vi "CSM Example - Caller is a CSM.vi"() -> ()   [LabVIEW 2017]
doc: "### CSM Example - Caller is a CSM.vi\n\n#### Overview\n\nDemonstrates how to invoke CSM module within the CSM framework. In this example, inter-module communication is performed through message string queue operations. You can generate a message string using the Build Message with Arguments++ VI or directly use message description strings if you are familiar with the format.\n\nThis example synchronously calls two instances of CSM Reuse Module.vi, enabling dynamic status subscription and module control through the API.\n\n#### Introduction\n\nDemonstrates how to invoke CSM module within the CSM framework. In this example, inter-module communication is performed through message string queue operations. You can generate a message string using the Build Message with Arguments++ VI or directly use message description strings if you are familiar with the format.\n\nThis example synchronously calls two instances of CSM Reuse Module.vi, enabling dynamic status subscription and module control through the API.\n\n#### Steps\n\nStep 1: Drop a VI CSM UI Module Template from LabVIEW palette, change the CSM name to \"CSMScenarioExample\".\n\nStep 2: Synchronously call the CSM Reuse Module.vi twice and name them SubModule0 and SubModule1 respectively. For more details of how to create such a reuse CSM module, please refer to another CSM-example named 1. Create a reuse Module.\n\nStep 3: Add one new line of customized message string, namely \"Macro: Switch Active Module\" as the last line into the existing standard string queues under \"Macro:Initialize\" case, so that we can switch between different SubModules.\n\nStep 4: Add one string constant SubModule0 for internal data initialization. For more customized internal data initialization, we can add more code here. \n\nStep 5: Add one string control in the UI to switch and display active/target module (Combox box).\n Step 5.1: Under \" 'Target Module': Value Change\" UI event, set the string control to the active module internal data and also send one intra-module message Macro: Switch Active. Module. \n Step 5.2: Under \"UI: Initialize\" case, update the active/Target Module.\n\nStep 6: Under \"Macro: Switch Active Module\" case, use the high level VI to send an inter-module sync. message \"API: Get Level -@ modulename\" to the active SubModule.\nOr you can also just type the string constant manually if you're familiar with the CSM string syntax rules. \n\nStep 7: Now the status queue is empty and the CSM state machine is now waiting in the timeout UI-event under ' \"\", \"Event Structure\", \"Idle\" '. The next step depends on the UI interaction provided by the User. \n\nStep 8: Create local test buttons/controls in the UI as follows:\n Step 8.1: Create API:Start button, when user clicks this button, a async-No reply message, \"API: Start -> modulename\" will be send to start the active subModule. \n Step 8.2: Create Register All Status Change button, when user clicks this button, this CSM module registers following broadcast/interrupt message from the active SubModule \n\"Status Changed@* >> Action: Status Change Handler -><register>\".\n Step 8.3: Create Unregister All Status Change button, when user clicks this button, this CSM module unregisters following broadcast/interrupt message from the active SubModule \n\"Status Changed@* >> Action: Status Change Handler -><unregister>\".\n Step 8.4: No code here, but you can see the log when it's called because of the registered status change. Any further customized code can be added here right after receiving this broadcast/interrupt message.\n Step 8.5: Create API:Stop button, when user clicks this button, an async-No reply message, \"API: Stop -> modulename\" will be sent to stop the active subModule. \n Step 8.6: Create Level DBL control, when user changes the value, an async message, \"API: Set Level >> 0.3 ->| modulename\" will be sent to the active subModule.\n Step 8.7: Create API: Get Level(Async) button, when user clicks this button, an async message, \"API: Get Level -> modulename\" will be sent to the active SubModule. Handle the case \"Async Message Posted\" and \"Async Response\" accordingly, in this example the Level display will be updated. \n Step 8.8: Create UI: create Front Panel State >> Open button, when user clicks the button, an async message with no reply \"UI: Front Panel State >> Open ->| modulename\" will be sent to the active Submodule.\n Step 8.9: Create UI: create Front Panel State >> Close button, when user clicks the button, an async message with no reply \"UI: Front Panel State >> Close ->| modulename\" will be sent to the active Submodule.\n\nStep 9: Under \"Panel Close?\" UI event, add two more new string messages before \"Macro:Exit\": \"Macro: Exit -@ SubModule0\" and \"Macro: Exit -@ SubModule1\", so that we can safely close all the CSM submodules before we finally close the CSM caller/main module."
uses:
  user.lib/_NEVSTOP/Communicable State Machine(CSM)/_Polymophic/Build Asynchronous Message with Arguments.vi
  user.lib/_NEVSTOP/Communicable State Machine(CSM)/_Polymophic/Build No-Reply Asynchronous Message with Arguments.vi
  user.lib/_NEVSTOP/Communicable State Machine(CSM)/_Polymophic/Build Unregister Status Message.vi
  user.lib/_NEVSTOP/Communicable State Machine(CSM)/_Polymophic/Build Register Status Message.vi
  user.lib/_NEVSTOP/Communicable State Machine(CSM)/_Polymophic/Build Synchronous Message with Arguments.vi
  user.lib/_NEVSTOP/Communicable State Machine(CSM)/Communicable State Machine.lvlib
  1. Create a reuse Module/1. Create a reuse Module.lvlib
panel:
  in  "UI: Front Panel State >> Close":bool
  in  "UI: Front Panel State >> Open":bool
  in  "Level":dbl min=0.0 max=1.0 step=0.1
  in  "Target Module":string(combo)="SubModule0"
  in  "API: Stop":bool
  in  "API: Start":bool
  in  "Unregister All Status Change":bool
  in  "Register All Status Change":bool
  in  "API: Get Level(Async)":bool
  out "State History of Main":string
  # "#CSM-Example Overview\n\nDemonstrates how to invoke CSM module within the CSM framework. In this example, inter-module communication is performed through message string queue operations. You can generate a message string using the Build Message with Arguments++ VI or directly use message description strings if you are familiar with the format.\n\nThis example synchronously calls two instances of CSM Reuse Module.vi, enabling dynamic status subscription and module control through the API."
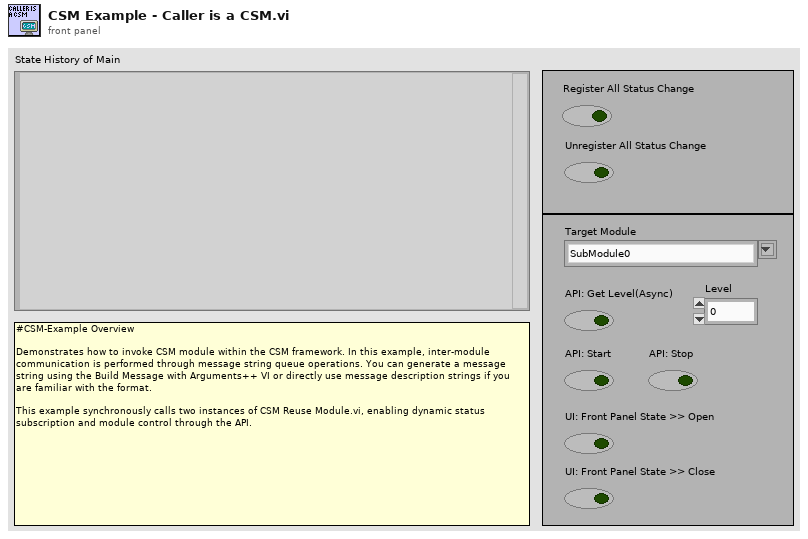
[diagram p1: front panel]
types:
  T1 = enum32{"Invalid", "Standard", "Closed", "Hidden", "Minimized", "Maximized"}
  T2 = enum32{"invalid app kind", "Development System", "Run Time System", "Student Edition", "Embedded LabVIEW", "Evaluation", "Custom"}
  T3 = typedef "Communicable State Machine.lvlib/_CSM_Response Source Message.ctl" = cluster{"‘State":string, "’Arguments":string, "’Error":errorcluster}
  T4 = cluster{"Core":cluster{"Current VI Reference":refnum<vi>, "Close Panel on Exit?":bool}, "Active Module":string}
  T5 = cluster{"Current VI Reference":refnum<vi>, "Close Panel on Exit?":bool}
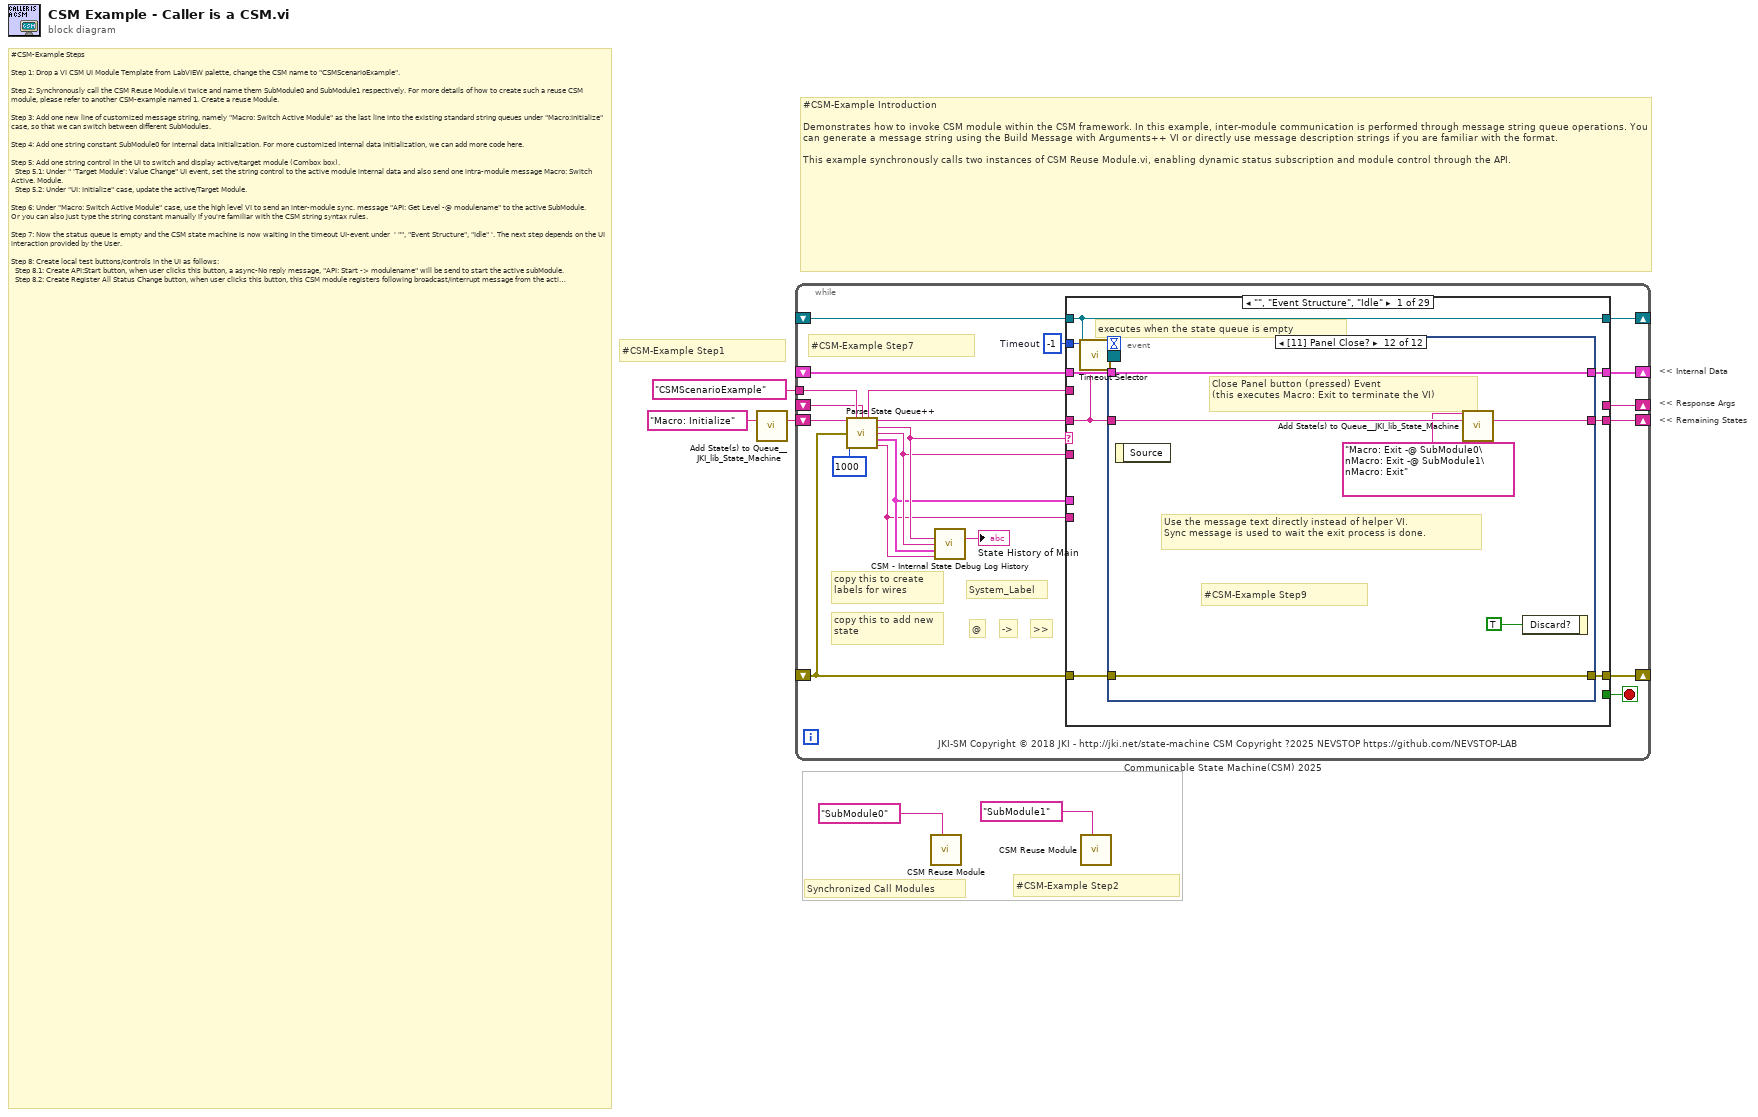
[diagram p0: block diagram]
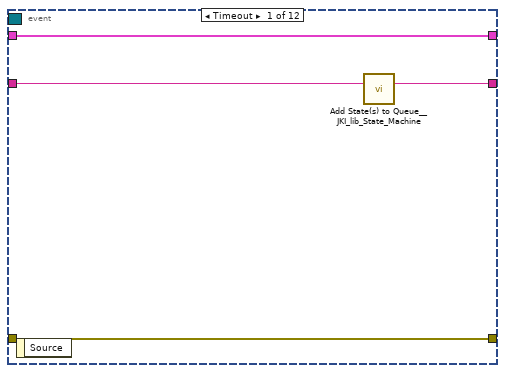
[diagram p2: hidden frame]
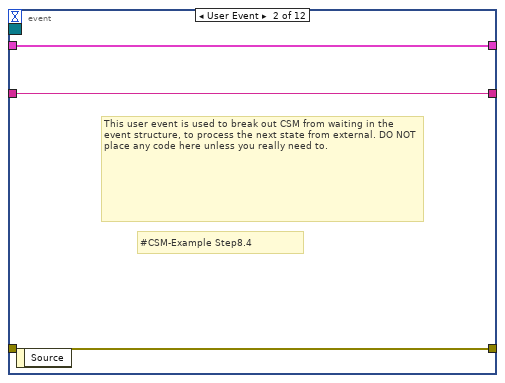
[diagram p3: hidden frame]
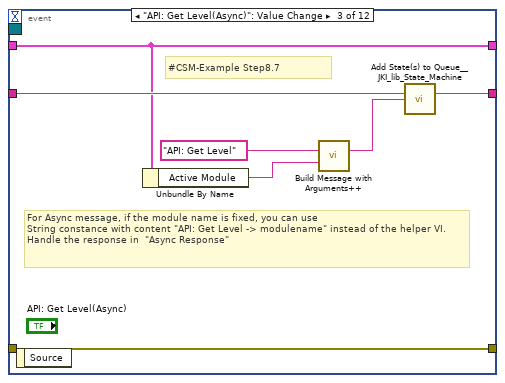
[diagram p4: hidden frame]
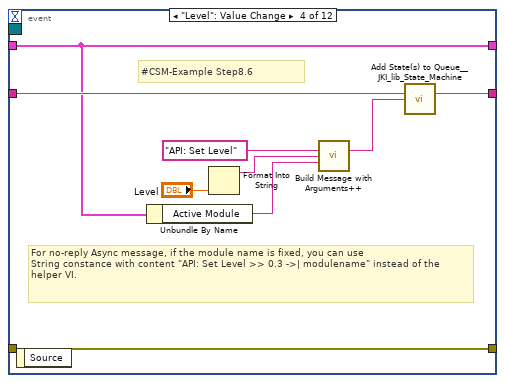
[diagram p5: hidden frame]
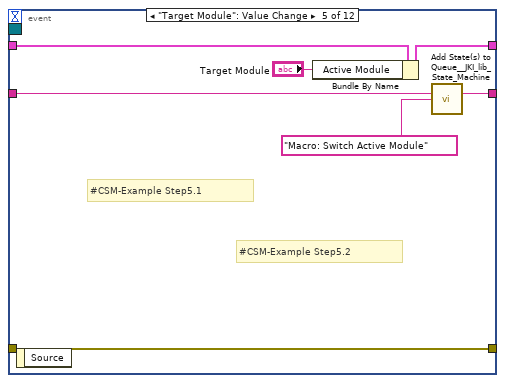
[diagram p6: hidden frame]
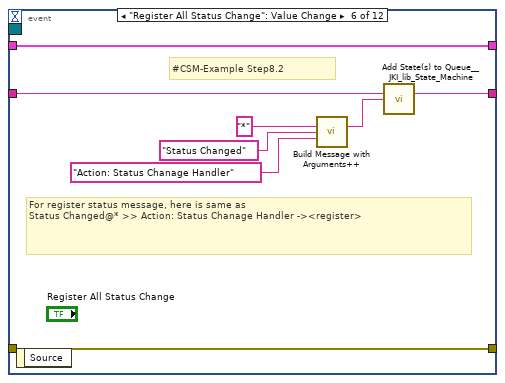
[diagram p7: hidden frame]
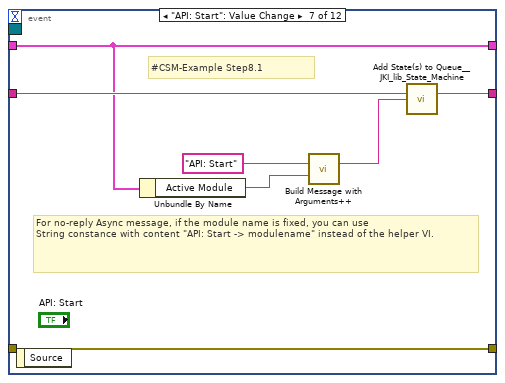
[diagram p8: hidden frame]
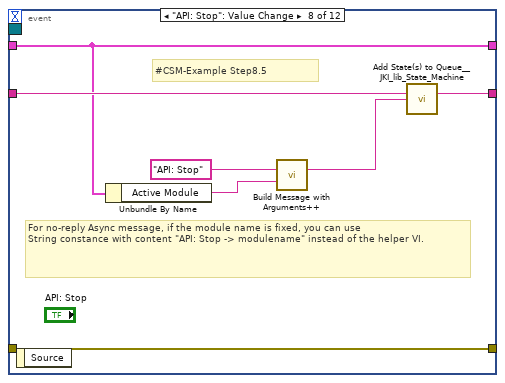
[diagram p9: hidden frame]
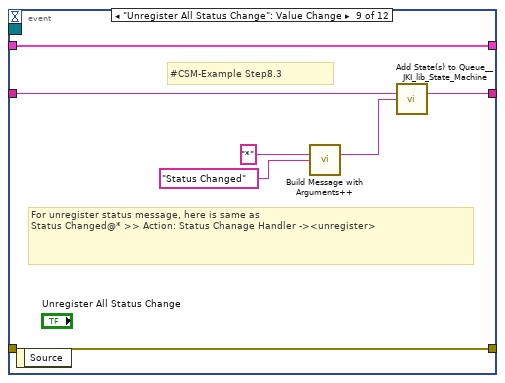
[diagram p10: hidden frame]
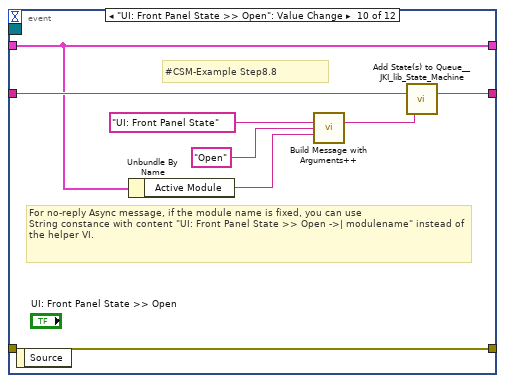
[diagram p11: hidden frame]
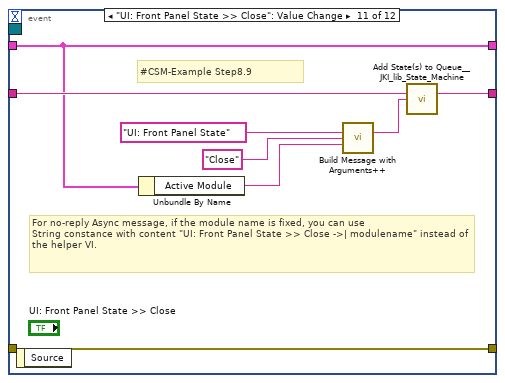
[diagram p12: hidden frame]
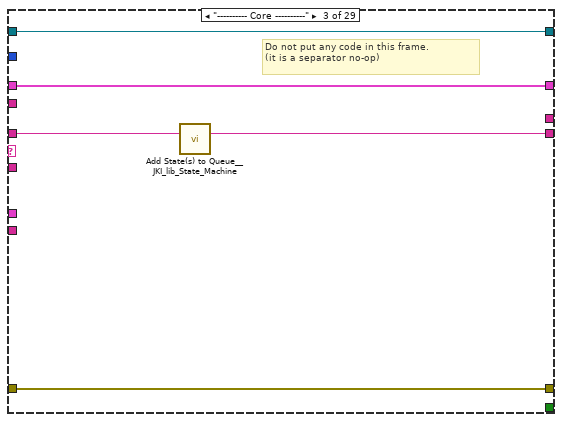
[diagram p14: hidden frame]
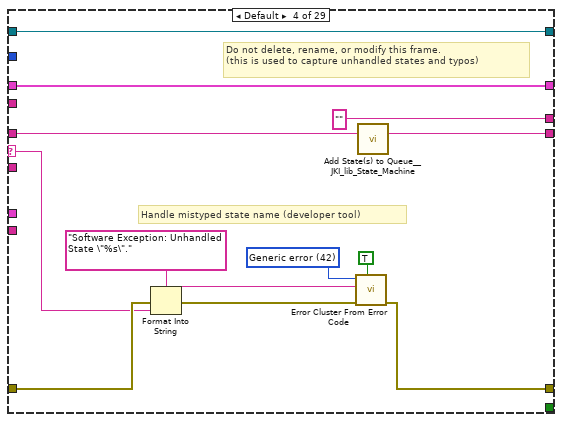
[diagram p15: hidden frame]
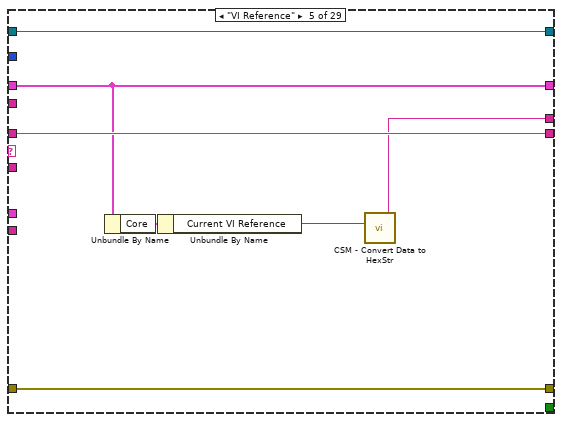
[diagram p16: hidden frame]
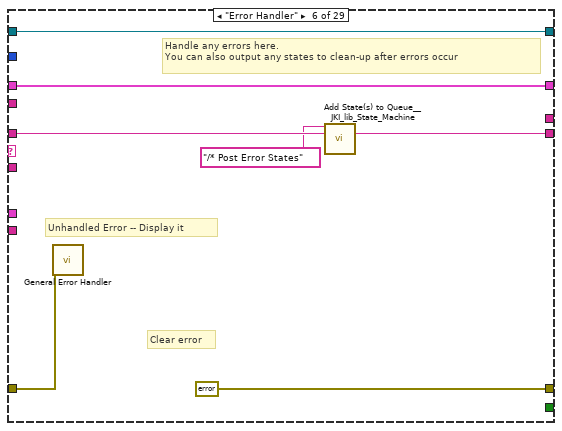
[diagram p17: hidden frame]
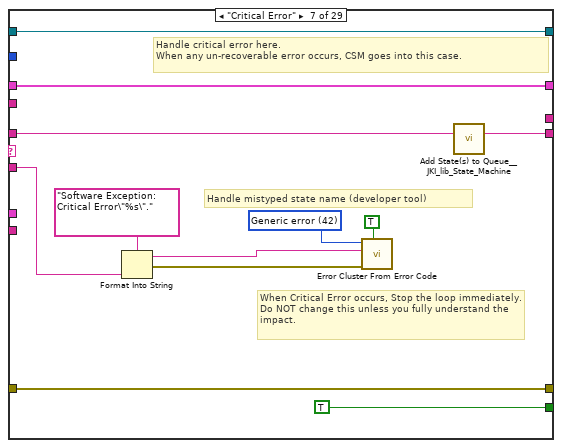
[diagram p18: hidden frame]
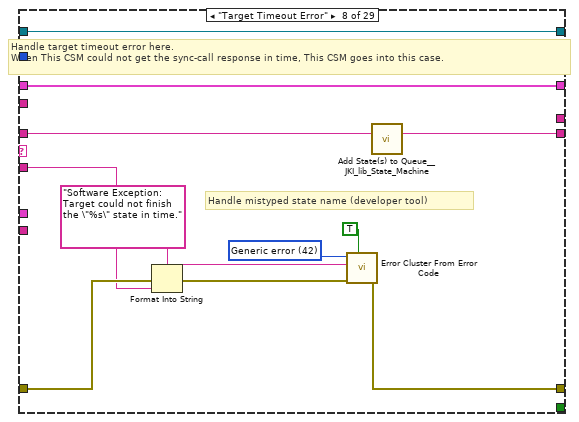
[diagram p19: hidden frame]
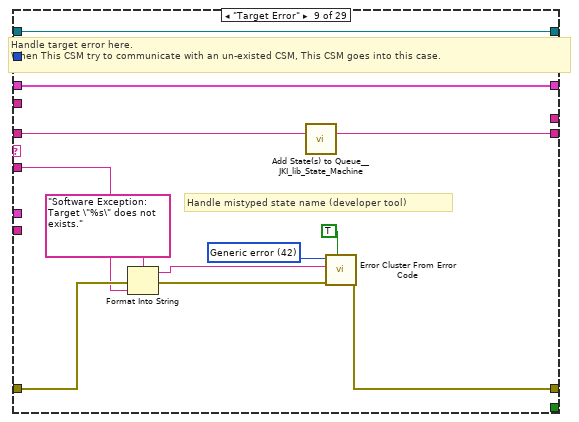
[diagram p20: hidden frame]
diagram:
  # "#CSM-Example Step2"
  # "#CSM-Example Step1"
  # "#CSM-Example Introduction\n\nDemonstrates how to invoke CSM module within the CSM framework. In this example, inter-module communication is performed through message string queue operations. You can generate a message string using the Build Message with Arguments++ VI or directly use message description strings if you are familiar with the format.\n\nThis example synchronously calls two instances of CSM Reuse Module.vi, enabling dynamic status subscription and module control through the API."
  # "#CSM-Example Steps\n\nStep 1: Drop a VI CSM UI Module Template from LabVIEW palette, change the CSM name to \"CSMScenarioExample\".\n\nStep 2: Synchronously call the CSM Reuse Module.vi twice and name them SubModule0 and SubModule1 respectively. For more details of how to create such a reuse CSM module, please refer to another CSM-example named 1. Create a reuse Module.\n\nStep 3: Add one new line of customized message string, namely \"Macro: Switch Active Module\" as the last line into the existing standard string queues under \"Macro:Initialize\" case, so that we can switch between different SubModules.\n\nStep 4: Add one string constant SubModule0 for internal data initialization. For more customized internal data initialization, we can add more code here. \n\nStep 5: Add one string control in the UI to switch and display active/target module (Combox box).\n  Step 5.1: Under \" 'Target Module': Value Change\" UI event, set the string control to the active module internal data and also send one intra-module message Macro: Switch Active. Module. \n  Step 5.2: Under \"UI: Initialize\" case, update the active/Target Module.\n\nStep 6: Under \"Macro: Switch Active Module\" case, use the high level VI to send an inter-module sync. message \"API: Get Level -@ modulename\" to the active SubModule.\nOr you can also just type the string constant manually if you're familiar with the CSM string syntax rules. \n\nStep 7: Now the status queue is empty and the CSM state machine is now waiting in the timeout UI-event under  ' \"\", \"Event Structure\", \"Idle\" '. The next step depends on the UI interaction provided by the User. \n\nStep 8: Create local test buttons/controls in the UI as follows:\n  Step 8.1: Create API:Start button, when user clicks this button, a async-No reply message, \"API: Start -> modulename\" will be send to start the active subModule. \n  Step 8.2: Create Register All Status Change button, when user clicks this button, this CSM module registers following broadcast/interrupt message from the active SubModule \n\"Status Changed@* >> Action: Status Change Handler -><register>\".\n  Step 8.3:  Create Unregister All Status Change button, when user clicks this button, this CSM module unregisters following broadcast/interrupt message from the active SubModule \n\"Status Changed@* >> Action: Status Change Handler -><unregister>\".\n  Step 8.4: No code here, but you can see the log when it's called because of the registered status change. Any further customized code can be added here right after receiving this broadcast/interrupt message.\n  Step 8.5: Create API:Stop button, when user clicks this button, an async-No reply message, \"API: Stop -> modulename\" will be sent to stop the active subModule. \n  Step 8.6: Create Level DBL control, when user changes the value, an async message, \"API: Set Level >> 0.3 ->| modulename\" will be sent to the active subModule.\n  Step 8.7: Create API: Get Level(Async) button, when user clicks this button, an async message, \"API: Get Level -> modulename\" will be sent to the active SubModule. Handle the case \"Async Message Posted\" and \"Async Response\" accordingly, in this example the Level display will be updated.  \n  Step 8.8: Create UI: create Front Panel State >> Open button, when user clicks the button, an async message with no reply \"UI: Front Panel State >> Open ->| modulename\" will be sent to the active Submodule.\n  Step 8.9: Create UI: create Front Panel State >> Close button, when user clicks the button, an async message with no reply \"UI: Front Panel State >> Close ->| modulename\" will be sent to the active Submodule.\n\nStep 9: Under \"Panel Close?\" UI event, add two more new string messages before \"Macro:Exit\": \"Macro: Exit -@ SubModule0\" and \"Macro: Exit -@ SubModule1\", so that we can safely close all the CSM submodules before we finally close the CSM caller/main module."
  # "Synchronized Call Modules"
  # "<< Internal Data"
  # "<< Response Args"
  # "<< Remaining States"
  n1 = call <vilib>:"Add State(s) to Queue__JKI_lib_State_Machine.vi"("State(s) in (\"\")"="Macro: Initialize") -> ("States Out"=w5:string)  [unwired: 14 in]
  n2 = while "Communicable State Machine(CSM) 2025" {
    shift-right: [w21] -> _
    shift-left: _ -> [w20]
    shift-right: [w24] -> _
    shift-left: _ -> [w18]
    shift-right: [w23] -> _
    shift-left: w5 -> [w25]
    tunnel: "CSMScenarioExample" ("Name (\"\" to Use UUID)") -> [w13]
    shift-right: [w16] -> _
    shift-left: _ -> [w7]
    shift-right: [w15] -> _
    shift-left: _ -> [w14]
    stop <- w22 stop-if-true
    w19 = -1  # Timeout
    # "#CSM-Example Step7"
    # "JKI-SM Copyright © 2018 JKI - http://jki.net/state-machine CSM Copyright ?2025 NEVSTOP https://github.com/NEVSTOP-LAB"
    # "copy this to add new state"
    # ">>"
    # "->"
    # "@"
    # "copy this to create labels for wires"
    # "System_Label"
    n3 = call "Parse State Queue++.vi"("State Queue"=w25, "Name (\"\" to Use UUID)"=w13, "Response Arguments"=w7, "Previous Error"=w18, "Response Timeout (-2 Use Global Settings)"=1000 ("Response Timeout(1000ms)")) -> ("Name Used"=w8:string, "Remaining States"=w26:string, "Current State"=w12:string, "Arguments"=w11:string, ">> Response Source Message >>"=w10:T3, ">> Source CSM >>"=w9:string)  [unwired: 5 in]
    n4 = call "CSM - Internal State Debug Log History.vi"("State"=w12, "Arguments (\"\")"=w11, ">> Response Source Message >>"=w10, "Source (\"\")"=w9) -> ("Debug Log"=→"State History of Main":string)  [unwired: 11 in]
    n5 = case shown="\"\", \"Event Structure\", \"Idle\"" w12 {
      selector: w12 -> [_ _ _ w128 _ _ _ _ _ _ _ _ _ _ _ _ _ _ _ _ _ _ _ _ _ _ _ _ _]
      tunnel: w26 -> [w27 w119 w125 w132 w144 w152 w162 w170 w182 w196 w202 w217 w223 w228 w235 w242 w247 w253 w257 w263 w269 w276 w288 w358 w364 w369 w383 w386 w390]
      tunnel: w11 -> [_ _ _ _ _ _ w155 w166 w178 w192 _ _ _ _ _ _ _ _ _ _ _ w271 w282 _ _ _ _ _ _]
      tunnel: w20 -> [w34 w118 w122 w130 w143 w149 w163 w168 w180 w195 w201 w210 w221 w225 _ w237 w244 w252 w256 w260 w265 w274 w284 w355 w361 w367 w380 w385 w389]
      tunnel: [w33 w120 w123 w134 w145 errorcluster {"status"=FALSE, "code"=0, "source"=""} ("error out") w164 w172 w184 w197 w203 w214 w220 w226 w232 w238 w245 w248 w255 w261 w267 w272 w285 w356 w362 w372 w381 w387 w391] -> w24
      tunnel: w18 -> [w32 w120 w123 w133 w145 w148 w164 w171 w183 w197 w203 w214 w220 w226 w232 w239 w245 _ w258 w261 w267 w273 w286 w356 w362 w372 w381 w387 w391]
      tunnel: [w35 w119 w124 w131 w144 w151 w161 w169 w181 w196 w202 w216 w222 w227 w234 w241 w246 w253 w257 w262 w268 w275 w287 w357 w363 w370 w382 w386 w390] -> w23
      tunnel: [_ _ _ _ _ _ TRUE _ _ _ _ _ TRUE _ _ _ _ _ _ _ _ _ _ _ _ _ _ _ _] -> w22
      tunnel: [w31 w118 w122 w130 w143 w149 w163 w168 w180 w195 w201 w215 w221 w225 w233 w237 w244 w252 w256 w260 w265 w274 w284 w355 w361 w367 w380 w385 w389] -> w21
      tunnel: w19 -> [w30 _ _ _ _ _ _ _ _ _ _ _ _ _ _ _ _ _ _ _ _ _ _ _ _ _ _ _ _]
      tunnel: w9 -> [_ _ _ _ _ _ _ _ _ w189 _ _ _ _ _ _ _ _ _ _ _ _ _ _ _ _ _ _ _]
      tunnel: w10 -> [_ _ _ _ _ _ _ _ _ w193 _ _ _ _ _ _ _ _ _ _ _ _ _ _ _ _ _ _ _]
      tunnel: [_ _ _ "" w139 _ _ _ _ _ _ _ _ _ _ _ _ _ _ _ _ _ _ _ _ _ _ _ _] -> w16
      tunnel: [w29 w117 w121 w126 w142 w146 w153 w165 w177 w194 w200 w204 w218 w224 w230 w236 w243 w251 w254 w259 w266 w270 w281 w354 w359 w371 w373 w384 w388] -> w15
      tunnel: w14 -> [w29 w117 w121 w126 w142 w146 w153 w165 w177 w194 w200 w204 w218 w224 w230 w236 w243 _ w254 w259 w266 w270 w281 w354 w359 w371 w373 w384 w388]
      tunnel: w8 -> [_ _ _ _ _ _ _ _ _ _ _ _ _ _ _ _ _ w250 _ _ _ _ _ _ _ _ _ _ _]
      frame "", "Event Structure", "Idle" {
        # "executes when the state queue is empty"
        n6 = call "Timeout Selector.vi"("Remaining States"=w27, "Timeout Expected"=w30) -> ("Timeout"=w28:i32)  [unwired: 5 in]
        n7 = event shown="[11] Panel Close?" {
          selector: w29 -> [_ _ _ _ _ _ _ _ _ _ _ _]
          dyn-events: _ -> [_ _ _ _ _ _ _ _ _ _ _ _]
          timeout: w28 -> [_ _ _ _ _ _ _ _ _ _ _ _]
          tunnel: w27 -> [w39 w41 w48 w57 w62 w71 w79 w86 w92 w101 w109 w116]
          tunnel: [w38 w41 w47 w56 w63 w70 w78 w85 w91 w100 w108 w115] -> w35
          tunnel: w34 -> [w36 w42 w44 w51 w64 w72 w75 w82 w93 w99 w106 w113]
          tunnel: [w37 w40 w49 w58 w65 w73 w80 w87 w94 w102 w110 w114] -> w33
          tunnel: w32 -> [w37 w40 w49 w58 w65 w73 w80 w87 w94 w102 w110 w114]
          tunnel: [w36 w42 w44 w51 w60 w72 w75 w82 w93 w99 w106 w113] -> w31
          event Timeout {
            n8 = event-data() -> ()  [unwired: 1 in, 1 out]
            n9 = call <vilib>:"Add State(s) to Queue__JKI_lib_State_Machine.vi"("State(s) in (\"\")"=w39) -> ("States Out"=w38:string)  [unwired: 14 in]
          }
          event User Event {
            # "#CSM-Example Step8.4"
            # "This user event is used to break out CSM from waiting in the event structure, to process the next state from external. DO NOT place any code here unless you really need to."
            n10 = event-data() -> ()  [unwired: 1 in, 1 out]
          }
          event "API: Get Level(Async)": Value Change {
            # "#CSM-Example Step8.7"
            # "For Async message, if the module name is fixed, you can use\nString constance with content \"API: Get Level -> modulename\" instead of the helper VI.  Handle the response in  \"Async Response\""
            n11 = event-data() -> ()  [unwired: 1 in, 1 out]
            n12 = Unbundle By Name(w44) -> ("Active Module"=w43:string)
            n13 = call-poly "Build Message with Arguments++.vi"("State With Arguments"="API: Get Level" ("State(s) in Front (\"\")"), "Target Module (\"\")"=w43) -> ("CSM Message String"=w45:string)  [unwired: 13 in]
            n14 = call <vilib>:"Add State(s) to Queue__JKI_lib_State_Machine.vi"("State(s) in (\"\")"=w48, "State(s) at Back (\"\")"=w45) -> ("States Out"=w47:string)  [unwired: 13 in]
          }
          event "Level": Value Change {
            # "#CSM-Example Step8.6"
            # "For no-reply Async message, if the module name is fixed, you can use\nString constance with content \"API: Set Level >> 0.3 ->| modulename\" instead of the helper VI."
            n15 = event-data() -> ()  [unwired: 1 in, 1 out]
            n16 = Unbundle By Name(w51) -> ("Active Module"=w50:string)
            n17 = Format Into String("Level") -> (resulting string=w52:string)  [unwired: 3 in, 1 out]
            n18 = call-poly "Build Message with Arguments++.vi"("State With Arguments"="API: Set Level" ("State(s) in Front (\"\")"), "Arguments (\"\")"=w52, "Target Module (\"\")"=w50) -> ("CSM Message String"=w54:string)  [unwired: 12 in]
            n19 = call <vilib>:"Add State(s) to Queue__JKI_lib_State_Machine.vi"("State(s) in (\"\")"=w57, "State(s) at Back (\"\")"=w54) -> ("States Out"=w56:string)  [unwired: 13 in]
          }
          event "Target Module": Value Change {
            # "#CSM-Example Step5.2"
            # "#CSM-Example Step5.1"
            n20 = event-data() -> ()  [unwired: 1 in, 1 out]
            n21 = Bundle By Name(cluster=w64, "Active Module"="Target Module") -> (w60:T4)
            n22 = call <vilib>:"Add State(s) to Queue__JKI_lib_State_Machine.vi"("State(s) in (\"\")"=w62, "State(s) at Back (\"\")"="Macro: Switch Active Module" ("State(s) at Back (\"\")")) -> ("States Out"=w63:string)  [unwired: 13 in]
          }
          event "Register All Status Change": Value Change {
            # "#CSM-Example Step8.2"
            # "For register status message, here is same as \nStatus Changed@* >> Action: Status Chanage Handler -><register>"
            n23 = event-data() -> ()  [unwired: 1 in, 1 out]
            n24 = call-poly "Build Message with Arguments++.vi"("Source CSM (* as Default)"="*" ("Source CSM Name (* as Default)"), "Status"="Status Changed", "API (If \"\", Same As \"Status\")"="Action: Status Chanage Handler" ("Status")) -> ("CSM Message String"=w66:string)  [unwired: 12 in]
            n25 = call <vilib>:"Add State(s) to Queue__JKI_lib_State_Machine.vi"("State(s) in (\"\")"=w71, "State(s) at Back (\"\")"=w66) -> ("States Out"=w70:string)  [unwired: 13 in]
          }
          event "API: Start": Value Change {
            # "#CSM-Example Step8.1"
            # "For no-reply Async message, if the module name is fixed, you can use\nString constance with content \"API: Start -> modulename\" instead of the helper VI."
            n26 = event-data() -> ()  [unwired: 1 in, 1 out]
            n27 = Unbundle By Name(w75) -> ("Active Module"=w74:string)
            n28 = call-poly "Build Message with Arguments++.vi"("State With Arguments"="API: Start" ("State(s) in Front (\"\")"), "Target Module (\"\")"=w74) -> ("CSM Message String"=w76:string)  [unwired: 13 in]
            n29 = call <vilib>:"Add State(s) to Queue__JKI_lib_State_Machine.vi"("State(s) in (\"\")"=w79, "State(s) at Back (\"\")"=w76) -> ("States Out"=w78:string)  [unwired: 13 in]
          }
          event "API: Stop": Value Change {
            # "#CSM-Example Step8.5"
            # "For no-reply Async message, if the module name is fixed, you can use\nString constance with content \"API: Stop -> modulename\" instead of the helper VI."
            n30 = event-data() -> ()  [unwired: 1 in, 1 out]
            n31 = Unbundle By Name(w82) -> ("Active Module"=w81:string)
            n32 = call-poly "Build Message with Arguments++.vi"("State With Arguments"="API: Stop" ("State(s) in Front (\"\")"), "Target Module (\"\")"=w81) -> ("CSM Message String"=w83:string)  [unwired: 13 in]
            n33 = call <vilib>:"Add State(s) to Queue__JKI_lib_State_Machine.vi"("State(s) in (\"\")"=w86, "State(s) at Back (\"\")"=w83) -> ("States Out"=w85:string)  [unwired: 13 in]
          }
          event "Unregister All Status Change": Value Change {
            # "#CSM-Example Step8.3"
            # "For unregister status message, here is same as \nStatus Changed@* >> Action: Status Chanage Handler -><unregister>"
            n34 = event-data() -> ()  [unwired: 1 in, 1 out]
            n35 = call-poly "Build Message with Arguments++.vi"("Source CSM (* as Default)"="*" ("Source CSM Name (* as Default)"), "Status"="Status Changed") -> ("CSM Message String"=w88:string)  [unwired: 13 in]
            n36 = call <vilib>:"Add State(s) to Queue__JKI_lib_State_Machine.vi"("State(s) in (\"\")"=w92, "State(s) at Back (\"\")"=w88) -> ("States Out"=w91:string)  [unwired: 13 in]
          }
          event "UI: Front Panel State >> Open": Value Change {
            # "#CSM-Example Step8.8"
            # "For no-reply Async message, if the module name is fixed, you can use\nString constance with content \"UI: Front Panel State >> Open ->| modulename\" instead of the helper VI."
            n37 = event-data() -> ()  [unwired: 1 in, 1 out]
            n38 = Unbundle By Name(w99) -> ("Active Module"=w98:string)
            n39 = call-poly "Build Message with Arguments++.vi"("State With Arguments"="UI: Front Panel State" ("CSM Name"), "Arguments (\"\")"="Open" ("CSM Name"), "Target Module (\"\")"=w98) -> ("CSM Message String"=w97:string)  [unwired: 12 in]
            n40 = call <vilib>:"Add State(s) to Queue__JKI_lib_State_Machine.vi"("State(s) in (\"\")"=w101, "State(s) at Back (\"\")"=w97) -> ("States Out"=w100:string)  [unwired: 13 in]
          }
          event "UI: Front Panel State >> Close": Value Change {
            # "#CSM-Example Step8.9"
            # "For no-reply Async message, if the module name is fixed, you can use\nString constance with content \"UI: Front Panel State >> Close ->| modulename\" instead of the helper VI."
            n41 = event-data() -> ()  [unwired: 1 in, 1 out]
            n42 = Unbundle By Name(w106) -> ("Active Module"=w105:string)
            n43 = call-poly "Build Message with Arguments++.vi"("State With Arguments"="UI: Front Panel State" ("CSM Name"), "Arguments (\"\")"="Close" ("CSM Name"), "Target Module (\"\")"=w105) -> ("CSM Message String"=w104:string)  [unwired: 12 in]
            n44 = call <vilib>:"Add State(s) to Queue__JKI_lib_State_Machine.vi"("State(s) in (\"\")"=w109, "State(s) at Back (\"\")"=w104) -> ("States Out"=w108:string)  [unwired: 13 in]
          }
          event Panel Close? {
            # "#CSM-Example Step9"
            # "Use the message text directly instead of helper VI.\nSync message is used to wait the exit process is done."
            # "Close Panel button (pressed) Event\n(this executes Macro: Exit to terminate the VI)"
            n45 = event-data() -> ()  [unwired: 1 in, 1 out]
            n46 = call <vilib>:"Add State(s) to Queue__JKI_lib_State_Machine.vi"("State(s) in Front (\"\")"="Macro: Exit -@ SubModule0\nMacro: Exit -@ SubModule1\nMacro: Exit", "State(s) in (\"\")"=w116) -> ("States Out"=w115:string)  [unwired: 13 in]
            n47 = event-data("Discard?"=TRUE) -> ()  [unwired: 1 in, 1 out]
          }
        }
      }
      frame "CSM Documentation" {
        # "#CSM README FIRST\n\nCSM is a LabVIEW application framework that builds upon JKI State Machine (JKISM). It follows the pattern of JKISM and extends the keywords to describe message communication between CSM modules, including concepts such as Sync-Message, Async-Message, Subscription/Unsubscription of status - essential elements for creating reusable code modules. For more information, please visit the CSM wiki: https://github.com/NEVSTOP-LAB/JKI-State-Machine-Plus-Plus/wiki\n\nFor instructions on JKI State Machine, visit: http://jki.net/state-machine/\nFor information about CSM, visit: https://github.com/NEVSTOP-LAB"
        # "CSM Documentation"
      }
      frame "---------- Core ----------" {
        # "Do not put any code in this frame.\n(it is a separator no-op)"
        n48 = call <vilib>:"Add State(s) to Queue__JKI_lib_State_Machine.vi"("State(s) in (\"\")"=w125) -> ("States Out"=w124:string)  [unwired: 14 in]
      }
      frame Default {
        w137 = 42 items=["No error", "Argument error", "Memory is full", "Out of zone", "End of file", "File already open", "Generic file I/O error", "File not found", "File permission error", "Disk is full", "Duplicate path", "Too many files open", "System feature not enabled", "Resource file not found", "Cannot add resource", "Resource not found", "Image not found", "Image memory error", "Pen does not exist", "Config type invalid", "Config token not found", "Config parse error", "Config memory error", "Bad external code format", "Bad external code offset", "External code not present", "Null window", "Destroy window error", "Null menu", "Print aborted", "Bad print record", "Print driver error", "Windows error during printing", "Memory error during printing", "Print dialog error", "Generic print error", "Invalid device refnum", "Device not found", "Device parameter error", "Device unit error", "Cannot open device", "Device call aborted", "Generic error", "Cancelled by user", "Object ID too low", "Object ID too high", "Object not in heap", "Unknown heap", "Unknown object (invalid DefProc)", "Unknown object (DefProc not in table)", "Message out of range", "Invalid (null) method", "Unknown message", "Manager call not supported", "Bad address", "Network operation in progress", "Network operation timed out", "Connection is busy", "Network attribute not supported", "Network error", "Address in use", "System out of memory", "Connection aborted", "Connection refused", "Not connected", "Already connected", "Connection closed", "Initialization error (interapplication manager)", "Bad occurrence", "Wait on unbound occurrence handler", "Occurrence queue overflow", "Datalog type conflict", "Unused", "Unrecognized type (interapplication manager)", "Memory corrupt", "Failed to make temporary DLL", "Old CIN version", "Drag socket not found", "Failed to load drop-object", "Failed to register OLE object", "Failed to release OLE object", "Format specifier type mismatch", "Unknown format specifier", "Too few format specifiers", "Too many format specifiers", "Scan failed", "Newer CIN version", "Error converting to variant", "Runtime menu error", "Password tampered", "Variant attribute not found", "Incompatible variant data type", "Event data is not available", "Event Store is not present", "Occurrence is not found", "Event Queue is not created", "Event info is not available", "Refnum passed is NULL", "Error retrieving Class GUID", "Error retrieving CoClass GUID", "Error retrieving TypeLib GUID.", "Bad built application magic bytes.", "Specific driver is different from the specific driver associated with the Logical Name.", "There is no session opened to the class driver.", "Max Error", "MAX - Error with config objects", "MAX - Error loading configuration", "MAX - Group not supported"]
        # "Do not delete, rename, or modify this frame.\n(this is used to capture unhandled states and typos)"
        # "Handle mistyped state name (developer tool)"
        n49 = Format Into String(format string="Software Exception: Unhandled State \"%s\"." ("message"), error in=w133, w128) -> (resulting string=w136:string, error out=w135:errorcluster)  [unwired: 1 in]
        n50 = call <vilib>:"Error Cluster From Error Code.vi"("show call chain? (False)"=TRUE, "error in (no error)"=w135, "error message (\"\")"=w136, "error code (0)"=w137) -> ("error out"=w134:errorcluster)  [unwired: 5 in]
        n51 = call <vilib>:"Add State(s) to Queue__JKI_lib_State_Machine.vi"("State(s) in (\"\")"=w132) -> ("States Out"=w131:string)  [unwired: 14 in]
      }
      frame "VI Reference" {
        n52 = Unbundle By Name(w143) -> ("Core"=w141:T5)
        n53 = Unbundle By Name(w141) -> ("Current VI Reference"=w140:refnum<vi>)
        n54 = call "CSM - Convert Data to HexStr.vi"("Variant"=w140) -> ("HEX String (0-9,A-F)"=w139:string)  [unwired: 8 in]
      }
      frame "Error Handler" {
        # "Unhandled Error -- Display it"
        # "Handle any errors here.\nYou can also output any states to clean-up after errors occur"
        # "Clear error"
        n55 = call <vilib>:"General Error Handler.vi"("error in (no error)"=w148) -> ()  [unwired: 10 in, 5 out]
        n56 = call <vilib>:"Add State(s) to Queue__JKI_lib_State_Machine.vi"("State(s) in Front (\"\")"="/* Post Error States", "State(s) in (\"\")"=w152) -> ("States Out"=w151:string)  [unwired: 13 in]
      }
      frame "Critical Error" {
        w159 = 42 items=["No error", "Argument error", "Memory is full", "Out of zone", "End of file", "File already open", "Generic file I/O error", "File not found", "File permission error", "Disk is full", "Duplicate path", "Too many files open", "System feature not enabled", "Resource file not found", "Cannot add resource", "Resource not found", "Image not found", "Image memory error", "Pen does not exist", "Config type invalid", "Config token not found", "Config parse error", "Config memory error", "Bad external code format", "Bad external code offset", "External code not present", "Null window", "Destroy window error", "Null menu", "Print aborted", "Bad print record", "Print driver error", "Windows error during printing", "Memory error during printing", "Print dialog error", "Generic print error", "Invalid device refnum", "Device not found", "Device parameter error", "Device unit error", "Cannot open device", "Device call aborted", "Generic error", "Cancelled by user", "Object ID too low", "Object ID too high", "Object not in heap", "Unknown heap", "Unknown object (invalid DefProc)", "Unknown object (DefProc not in table)", "Message out of range", "Invalid (null) method", "Unknown message", "Manager call not supported", "Bad address", "Network operation in progress", "Network operation timed out", "Connection is busy", "Network attribute not supported", "Network error", "Address in use", "System out of memory", "Connection aborted", "Connection refused", "Not connected", "Already connected", "Connection closed", "Initialization error (interapplication manager)", "Bad occurrence", "Wait on unbound occurrence handler", "Occurrence queue overflow", "Datalog type conflict", "Unused", "Unrecognized type (interapplication manager)", "Memory corrupt", "Failed to make temporary DLL", "Old CIN version", "Drag socket not found", "Failed to load drop-object", "Failed to register OLE object", "Failed to release OLE object", "Format specifier type mismatch", "Unknown format specifier", "Too few format specifiers", "Too many format specifiers", "Scan failed", "Newer CIN version", "Error converting to variant", "Runtime menu error", "Password tampered", "Variant attribute not found", "Incompatible variant data type", "Event data is not available", "Event Store is not present", "Occurrence is not found", "Event Queue is not created", "Event info is not available", "Refnum passed is NULL", "Error retrieving Class GUID", "Error retrieving CoClass GUID", "Error retrieving TypeLib GUID.", "Bad built application magic bytes.", "Specific driver is different from the specific driver associated with the Logical Name.", "There is no session opened to the class driver.", "Max Error", "MAX - Error with config objects", "MAX - Error loading configuration", "MAX - Group not supported"]
        # "Handle critical error here.\nWhen any un-recoverable error occurs, CSM goes into this case."
        # "When Critical Error occurs, Stop the loop immediately. Do NOT change this unless you fully understand the impact."
        # "Handle mistyped state name (developer tool)"
        n57 = Format Into String(format string="Software Exception: Critical Error\"%s\"." ("message"), w155) -> (resulting string=w158:string, error out=w157:errorcluster)  [unwired: 2 in]
        n58 = call <vilib>:"Error Cluster From Error Code.vi"("show call chain? (False)"=TRUE, "error in (no error)"=w157, "error message (\"\")"=w158, "error code (0)"=w159) -> ()  [unwired: 5 in, 1 out]
        n59 = call <vilib>:"Add State(s) to Queue__JKI_lib_State_Machine.vi"("State(s) in (\"\")"=w162) -> ("States Out"=w161:string)  [unwired: 14 in]
      }
      frame "Target Timeout Error" {
        w175 = 42 items=["No error", "Argument error", "Memory is full", "Out of zone", "End of file", "File already open", "Generic file I/O error", "File not found", "File permission error", "Disk is full", "Duplicate path", "Too many files open", "System feature not enabled", "Resource file not found", "Cannot add resource", "Resource not found", "Image not found", "Image memory error", "Pen does not exist", "Config type invalid", "Config token not found", "Config parse error", "Config memory error", "Bad external code format", "Bad external code offset", "External code not present", "Null window", "Destroy window error", "Null menu", "Print aborted", "Bad print record", "Print driver error", "Windows error during printing", "Memory error during printing", "Print dialog error", "Generic print error", "Invalid device refnum", "Device not found", "Device parameter error", "Device unit error", "Cannot open device", "Device call aborted", "Generic error", "Cancelled by user", "Object ID too low", "Object ID too high", "Object not in heap", "Unknown heap", "Unknown object (invalid DefProc)", "Unknown object (DefProc not in table)", "Message out of range", "Invalid (null) method", "Unknown message", "Manager call not supported", "Bad address", "Network operation in progress", "Network operation timed out", "Connection is busy", "Network attribute not supported", "Network error", "Address in use", "System out of memory", "Connection aborted", "Connection refused", "Not connected", "Already connected", "Connection closed", "Initialization error (interapplication manager)", "Bad occurrence", "Wait on unbound occurrence handler", "Occurrence queue overflow", "Datalog type conflict", "Unused", "Unrecognized type (interapplication manager)", "Memory corrupt", "Failed to make temporary DLL", "Old CIN version", "Drag socket not found", "Failed to load drop-object", "Failed to register OLE object", "Failed to release OLE object", "Format specifier type mismatch", "Unknown format specifier", "Too few format specifiers", "Too many format specifiers", "Scan failed", "Newer CIN version", "Error converting to variant", "Runtime menu error", "Password tampered", "Variant attribute not found", "Incompatible variant data type", "Event data is not available", "Event Store is not present", "Occurrence is not found", "Event Queue is not created", "Event info is not available", "Refnum passed is NULL", "Error retrieving Class GUID", "Error retrieving CoClass GUID", "Error retrieving TypeLib GUID.", "Bad built application magic bytes.", "Specific driver is different from the specific driver associated with the Logical Name.", "There is no session opened to the class driver.", "Max Error", "MAX - Error with config objects", "MAX - Error loading configuration", "MAX - Group not supported"]
        # "Handle target timeout error here.\nWhen This CSM could not get the sync-call response in time, This CSM goes into this case."
        # "Handle mistyped state name (developer tool)"
        n60 = Format Into String(format string="Software Exception: Target could not finish the \"%s\" state in time." ("message"), error in=w171, w166) -> (resulting string=w174:string, error out=w173:errorcluster)  [unwired: 1 in]
        n61 = call <vilib>:"Error Cluster From Error Code.vi"("show call chain? (False)"=TRUE, "error in (no error)"=w173, "error message (\"\")"=w174, "error code (0)"=w175) -> ("error out"=w172:errorcluster)  [unwired: 5 in]
        n62 = call <vilib>:"Add State(s) to Queue__JKI_lib_State_Machine.vi"("State(s) in (\"\")"=w170) -> ("States Out"=w169:string)  [unwired: 14 in]
      }
      frame "Target Error" {
        w187 = 42 items=["No error", "Argument error", "Memory is full", "Out of zone", "End of file", "File already open", "Generic file I/O error", "File not found", "File permission error", "Disk is full", "Duplicate path", "Too many files open", "System feature not enabled", "Resource file not found", "Cannot add resource", "Resource not found", "Image not found", "Image memory error", "Pen does not exist", "Config type invalid", "Config token not found", "Config parse error", "Config memory error", "Bad external code format", "Bad external code offset", "External code not present", "Null window", "Destroy window error", "Null menu", "Print aborted", "Bad print record", "Print driver error", "Windows error during printing", "Memory error during printing", "Print dialog error", "Generic print error", "Invalid device refnum", "Device not found", "Device parameter error", "Device unit error", "Cannot open device", "Device call aborted", "Generic error", "Cancelled by user", "Object ID too low", "Object ID too high", "Object not in heap", "Unknown heap", "Unknown object (invalid DefProc)", "Unknown object (DefProc not in table)", "Message out of range", "Invalid (null) method", "Unknown message", "Manager call not supported", "Bad address", "Network operation in progress", "Network operation timed out", "Connection is busy", "Network attribute not supported", "Network error", "Address in use", "System out of memory", "Connection aborted", "Connection refused", "Not connected", "Already connected", "Connection closed", "Initialization error (interapplication manager)", "Bad occurrence", "Wait on unbound occurrence handler", "Occurrence queue overflow", "Datalog type conflict", "Unused", "Unrecognized type (interapplication manager)", "Memory corrupt", "Failed to make temporary DLL", "Old CIN version", "Drag socket not found", "Failed to load drop-object", "Failed to register OLE object", "Failed to release OLE object", "Format specifier type mismatch", "Unknown format specifier", "Too few format specifiers", "Too many format specifiers", "Scan failed", "Newer CIN version", "Error converting to variant", "Runtime menu error", "Password tampered", "Variant attribute not found", "Incompatible variant data type", "Event data is not available", "Event Store is not present", "Occurrence is not found", "Event Queue is not created", "Event info is not available", "Refnum passed is NULL", "Error retrieving Class GUID", "Error retrieving CoClass GUID", "Error retrieving TypeLib GUID.", "Bad built application magic bytes.", "Specific driver is different from the specific driver associated with the Logical Name.", "There is no session opened to the class driver.", "Max Error", "MAX - Error with config objects", "MAX - Error loading configuration", "MAX - Group not supported"]
        # "Handle target error here.\nWhen This CSM try to communicate with an un-existed CSM, This CSM goes into this case."
        # "Handle mistyped state name (developer tool)"
        n63 = Format Into String(format string="Software Exception: Target \"%s\" does not exists." ("message"), error in=w183, w178) -> (resulting string=w186:string, error out=w185:errorcluster)  [unwired: 1 in]
        n64 = call <vilib>:"Add State(s) to Queue__JKI_lib_State_Machine.vi"("State(s) in (\"\")"=w182) -> ("States Out"=w181:string)  [unwired: 14 in]
        n65 = call <vilib>:"Error Cluster From Error Code.vi"("show call chain? (False)"=TRUE, "error in (no error)"=w185, "error message (\"\")"=w186, "error code (0)"=w187) -> ("error out"=w184:errorcluster)  [unwired: 5 in]
      }
      frame "Async Response", "Response" {
        # "Handle Async-call Response (\"Async Response\" for ->)"
        # "Handle Sync-call Response (\"Response\" for @)"
        n66 = Unbundle(w193) -> ("‘State"=w191:string, "’Arguments"=w190:string)  [unwired: 1 out]
        n67 = case shown="\"False\", Default" w191 {
          tunnel: w192 -> [_ w199]
          tunnel: w190 -> [_ _]
          tunnel: w189 -> [_ _]
          frame "False", Default {
          }
          frame "API: Get Level" {
            n68 = Fract/Exp String To Number(string=w199) -> (number=w198:dbl)  [unwired: 3 in, 1 out]
            n69 = local write "Level"(w198) -> ()
          }
        }
      }
      frame "Async Message Posted" {
        # "Handle post action for async message (->)."
        # "After Async Message is posted (->), CSM goes to this state for post-action. You can use Argument - State to tell which Async Message is called."
      }
      frame "Initialize Core Data" {
        # "Do not delete, rename, or modify this frame.\n(this is used to determine panel behavior on exit)"
        # "originally closed?"
        # "exe?"
        # "If panel starts closed or is an EXE, then close it when we exit"
        n70 = property class="VI"() -> ("FP.State"=w207:T1)  [unwired: 2 in, 2 out]
        n71 = property class="App"() -> ("App.Kind"=w213:T2)  [unwired: 2 in, 2 out]
        n72 = control-ref of="Current VI Reference"() -> (w208:refnum<vi>)
        n73 = Equal?(x=w207, y=T1."Closed" ("Front Panel Window:State")) -> (x = y?=w205:bool)
        n74 = Equal?(x=w213, y=T2."Run Time System" ("Application:Kind")) -> (x = y?=w211:bool)
        n75 = Or(x=w205, y=w211) -> (x .or. y?=w209:bool)
        n76 = Bundle By Name(cluster=w210, "Core.Current VI Reference"=w208, "Core.Close Panel on Exit?"=w209) -> (w215:T4)
        n77 = call <vilib>:"Add State(s) to Queue__JKI_lib_State_Machine.vi"("State(s) in (\"\")"=w217) -> ("States Out"=w216:string)  [unwired: 14 in]
      }
      frame "Exit" {
        # "Do not put any code in this frame.\n(No errors that occur here will be handled.)"
        n78 = call <vilib>:"Add State(s) to Queue__JKI_lib_State_Machine.vi"("State(s) in (\"\")"=w223) -> ("States Out"=w222:string)  [unwired: 14 in]
      }
      frame "---------- Data ----------" {
        # "Do not put any code in this frame.\n(It is a separator no-op. You can make a copy of this frame to create a new Data frame)"
        n79 = call <vilib>:"Add State(s) to Queue__JKI_lib_State_Machine.vi"("State(s) in (\"\")"=w228) -> ("States Out"=w227:string)  [unwired: 14 in]
      }
      frame "Data: Initialize" {
        w229 = "SubModule0"  # Active Module
        w231 = T5 {"Current VI Reference"=refnum, "Close Panel on Exit?"=FALSE}  # Core
        # "#CSM-Example Step4"
        # "Initialize the shift-register data, here.\n(data names are defined by what you wire into the bundle function)"
        n80 = Bundle("Core"=w231, "Active Module"=w229) -> (w233:T4)  [unwired: 1 in]
        n81 = call <vilib>:"Add State(s) to Queue__JKI_lib_State_Machine.vi"("State(s) in (\"\")"=w235) -> ("States Out"=w234:string)  [unwired: 14 in]
      }
      frame "Data: Cleanup" {
        # "Cleanup any data and references, here.\n(this is called automatically, by the Macro: Exit)"
        n82 = Unbundle By Name(w237) -> ("Core.Current VI Reference"=w240:refnum<vi>)
        n83 = Close Reference(reference=w240, error in (no error)=w239) -> (error out=w238:errorcluster)
        n84 = call <vilib>:"Add State(s) to Queue__JKI_lib_State_Machine.vi"("State(s) in (\"\")"=w242) -> ("States Out"=w241:string)  [unwired: 14 in]
      }
      frame "---------- Events ----------" {
        # "Do not put any code in this frame.\n(It is a separator no-op. You can make a copy of this frame to create a new UI frame)"
        n85 = call <vilib>:"Add State(s) to Queue__JKI_lib_State_Machine.vi"("State(s) in (\"\")"=w247) -> ("States Out"=w246:string)  [unwired: 14 in]
      }
      frame "Events: Register" {
        # "Register message event to break Waiting in Event structure."
        n86 = call "CSM - Get New State Notifier Event.vi"("Name (\"\" to Use UUID) In"=w250) -> ("error out"=w248:errorcluster, "New State Notifier Event"=w249:refnum<user-event>)  [unwired: 9 in]
        n87 = register-events(w249) -> (reference out=w251:refnum<event-registration>)  [unwired: 2 in, 1 out]
      }
      frame "Events: Unregister" {
        n88 = Unregister For Events(event registration refnum=w254, error in=w258) -> (error out=w255:errorcluster)
      }
      frame "---------- UI ----------" {
        # "Do not put any code in this frame.\n(It is a separator no-op. You can make a copy of this frame to create a new UI frame)"
        n89 = call <vilib>:"Add State(s) to Queue__JKI_lib_State_Machine.vi"("State(s) in (\"\")"=w263) -> ("States Out"=w262:string)  [unwired: 14 in]
      }
      frame "UI: Initialize" {
        # "Initialize the User Interface, here.\n(this is called automatically, by the Macro: Init)"
        n90 = Unbundle By Name(w265) -> ("Active Module"=w264:string)
        n91 = local write "Target Module"(w264) -> ()
        n92 = call <vilib>:"Add State(s) to Queue__JKI_lib_State_Machine.vi"("State(s) in (\"\")"=w269) -> ("States Out"=w268:string)  [unwired: 14 in]
      }
      frame "UI: Cursor Set" {
        # "Argument"
        # "Set and Unset Cursor Busy.\n(Usage: \"UI: Cursor Set >> Busy|Idle\")"
        n93 = case shown="\"Idle\", Default" w271 {
          tunnel: w273 -> [w278 w280]
          tunnel: [w277 w279] -> w272
          frame "Idle", Default {
            n94 = call <vilib>:"Unset Busy.vi"("error in (no error)"=w278) -> ("error out"=w277:errorcluster)  [unwired: 10 in]
          }
          frame "Busy" {
            n95 = call <vilib>:"Set Busy.vi"("error in (no error)"=w280) -> ("error out"=w279:errorcluster)  [unwired: 9 in, 1 out]
          }
        }
        n96 = call <vilib>:"Add State(s) to Queue__JKI_lib_State_Machine.vi"("State(s) in (\"\")"=w276) -> ("States Out"=w275:string)  [unwired: 14 in]
      }
      frame "UI: Front Panel State" {
        # "Argument"
        # "Set Front Panel Open or Closed\n(Usage: \"UI: Front Panel State >> Open|Close\")"
        n97 = Unbundle By Name(w284) -> ("Core.Current VI Reference"=w283:refnum<vi>)
        n98 = call <vilib>:"Add State(s) to Queue__JKI_lib_State_Machine.vi"("State(s) in (\"\")"=w288) -> ("States Out"=w287:string)  [unwired: 14 in]
        n99 = case shown="\"Minimize\", \"Minimized\"" w282 {
          tunnel: w286 -> [w294 w309 w320 w333 w346]
          tunnel: [w296 w310 w322 w335 w348] -> w285
          tunnel: w283 -> [w295 w307 w321 w334 w347]
          frame "Open", "Standard", Default {
            w289 = T1."Standard" ("State")
            n100 = property class="VI"(reference=w295, error in=w294) -> (reference out=w292:refnum<vi>, error out=w293:errorcluster, "FP.State"=w291:T1)
            n101 = Not Equal?(x=w291, y=w289) -> (x != y?=w290:bool)
            n102 = case shown="True" w290 {
              tunnel: [w300 w302] -> w296
              tunnel: w293 -> [w299 w302]
              tunnel: w292 -> [w298 _]
              tunnel: w289 -> [w297 _]
              frame True {
                n103 = invoke class="VI" method="FP.Open"(reference=w298, error in=w299, "Activate"=TRUE, "State"=w297) -> (error out=w300:errorcluster)  [unwired: 1 in, 4 out]
              }
              frame False {
              }
            }
          }
          frame "Close", "Closed" {
            n104 = property class="VI"(reference=w307, error in=w309) -> (reference out=w306:refnum<vi>, error out=w308:errorcluster, "FP.State"=w304:T1)
            n105 = Not Equal?(x=w304, y=T1."Closed" ("Front Panel Window:State")) -> (x != y?=w303:bool)
            n106 = case shown="True" w303 {
              tunnel: [w311 w314] -> w310
              tunnel: w308 -> [w311 w313]
              tunnel: w306 -> [_ w312]
              frame False {
              }
              frame True {
                n107 = invoke class="VI" method="FP.Close"(reference=w312, error in=w313) -> (error out=w314:errorcluster)  [unwired: 1 in, 2 out]
              }
            }
          }
          frame "Hidden", "Hide" {
            w315 = T1."Hidden" ("State")
            n108 = property class="VI"(reference=w321, error in=w320) -> (reference out=w318:refnum<vi>, error out=w319:errorcluster, "FP.State"=w317:T1)
            n109 = Not Equal?(x=w317, y=w315) -> (x != y?=w316:bool)
            n110 = case shown="True" w316 {
              tunnel: [w326 w327] -> w322
              tunnel: w319 -> [w325 w327]
              tunnel: w318 -> [w324 _]
              tunnel: w315 -> [w323 _]
              frame True {
                n111 = invoke class="VI" method="FP.Open"(reference=w324, error in=w325, "State"=w323) -> (error out=w326:errorcluster)  [unwired: 2 in, 4 out]
              }
              frame False {
              }
            }
          }
          frame "Minimize", "Minimized" {
            w328 = T1."Minimized" ("State")
            n112 = property class="VI"(reference=w334, error in=w333) -> (reference out=w331:refnum<vi>, error out=w332:errorcluster, "FP.State"=w330:T1)
            n113 = Not Equal?(x=w330, y=w328) -> (x != y?=w329:bool)
            n114 = case shown="True" w329 {
              tunnel: [w339 w340] -> w335
              tunnel: w332 -> [w338 w340]
              tunnel: w331 -> [w337 _]
              tunnel: w328 -> [w336 _]
              frame True {
                n115 = invoke class="VI" method="FP.Open"(reference=w337, error in=w338, "State"=w336) -> (error out=w339:errorcluster)  [unwired: 2 in, 4 out]
              }
              frame False {
              }
            }
          }
          frame "Maximize", "Maximized" {
            w341 = T1."Maximized" ("State")
            n116 = property class="VI"(reference=w347, error in=w346) -> (reference out=w344:refnum<vi>, error out=w345:errorcluster, "FP.State"=w343:T1)
            n117 = Not Equal?(x=w343, y=w341) -> (x != y?=w342:bool)
            n118 = case shown="True" w342 {
              tunnel: [w352 w353] -> w348
              tunnel: w345 -> [w351 w353]
              tunnel: w344 -> [w350 _]
              tunnel: w341 -> [w349 _]
              frame True {
                n119 = invoke class="VI" method="FP.Open"(reference=w350, error in=w351, "State"=w349) -> (error out=w352:errorcluster)  [unwired: 2 in, 4 out]
              }
              frame False {
              }
            }
          }
        }
      }
      frame "---------- Macro ----------" {
        # "Do not put any code in this frame.\n(It is a separator no-op. You can make a copy of this frame to create a new Macro frame)"
        n120 = call <vilib>:"Add State(s) to Queue__JKI_lib_State_Machine.vi"("State(s) in (\"\")"=w358) -> ("States Out"=w357:string)  [unwired: 14 in]
      }
      frame "Macro: Initialize" {
        w360 = "Data: Initialize\nInitialize Core Data\nEvents: Register\nUI: Initialize\nUI: Front Panel State >> Open\nMacro: Switch Active Module"  # Data: Initialize Initialize Core Data Events: Register UI: Initialize UI: Front Panel State >> Open Macro: Switch Active Module
        # "#CSM-Example Step3"
        # "Initialization Macro\n(This is called once, when the VI starts)"
        n121 = call <vilib>:"Add State(s) to Queue__JKI_lib_State_Machine.vi"("State(s) in Front (\"\")"=w360, "State(s) in (\"\")"=w364) -> ("States Out"=w363:string)  [unwired: 13 in]
      }
      frame "Macro: Switch Active Module" {
        # "#CSM-Example Step6"
        # "For Sync message, if the module name is fixed, you can use\nString constance with content \"API: Get Level -@ modulename\" instead of the helper VI."
        n122 = Unbundle By Name(w367) -> ("Active Module"=w366:string)
        n123 = call-poly "Build Message with Arguments++.vi"("State With Arguments"="API: Get Level" ("State(s) in Front (\"\")"), "Target Module (\"\")"=w366) -> ("CSM Message String"=w365:string)  [unwired: 13 in]
        n124 = call <vilib>:"Add State(s) to Queue__JKI_lib_State_Machine.vi"("State(s) in Front (\"\")"=w365, "State(s) in (\"\")"=w369) -> ("States Out"=w370:string)  [unwired: 13 in]
      }
      frame "Macro: Exit" {
        # "Exit Macro\n(This is called once, when the VI exits)"
        n125 = Unbundle By Name(w380) -> ("Core.Close Panel on Exit?"=w379:bool)
        n126 = Select(t="UI: Front Panel State >> Close", s=w379, f="") -> (s? t:f=w376:string)
        n127 = call <vilib>:"Add State(s) to Queue__JKI_lib_State_Machine.vi"("State(s) in (\"\")"=w376, "State(s) at Back (\"\")"="Data: Cleanup\nEvents: Unregister\nExit") -> ("States Out"=w374:string)  [unwired: 13 in]
        n128 = call <vilib>:"Add State(s) to Queue__JKI_lib_State_Machine.vi"("State(s) in Front (\"\")"=w374, "State(s) in (\"\")"=w383) -> ("States Out"=w382:string)  [unwired: 13 in]
      }
      frame "------- Action -------" {
      }
      frame "Action: Status Chanage Handler" {
        # "No Code here. \nBut you can see the log when it's called because of the registered status change."
      }
    }
  }
  n129 = call "CSM Reuse Module.vi"("Name (\"\" to Use UUID)"="SubModule0" ("Name (\"\" to Use UUID)")) -> ()  [unwired: 11 in]
  n130 = call "CSM Reuse Module.vi"("Name (\"\" to Use UUID)"="SubModule1" ("Name (\"\" to Use UUID)")) -> ()  [unwired: 11 in]
